vi "移动鼠标并单击.vi"(8 "错误输入（无错误）":errorcluster, 10 "dy":i32=36, 11 "dx":i32=1683) -> (0 "错误输出":errorcluster)   [LabVIEW 2012]
uses:
  User32.dll
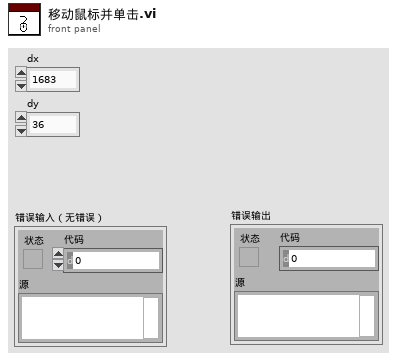
[diagram p1: front panel]
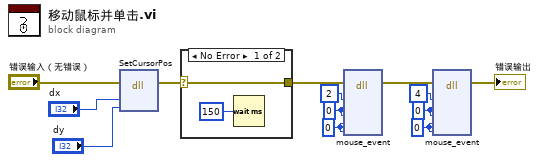
[diagram p0: block diagram]
diagram:
  w4 = 0 ("dwExtraInfo")
  w5 = u32 0 ("dwExtraInfo")
  w8 = 0 ("dwExtraInfo")
  w9 = u32 0 ("dwExtraInfo")
  n1 = dll-call lib="User32.dll" fn="SetCursorPos" ("Move mouse to new pos")(error in="错误输入（无错误）", "dx"="dx", "dy"="dy") -> (error out=w11:errorcluster)  [unwired: 5 in, 1 out]
  n2 = case shown="No Error" w11 {
    selector: w11 -> [w14 w16]
    tunnel: [w14 w16] -> w7
    frame No Error {
      n3 = Wait (ms)(milliseconds to wait=u32 150 ("等待时间（毫秒）")) -> ()  [unwired: 1 out]
    }
    frame Error {
    }
  }
  n4 = dll-call lib="user32.dll" fn="mouse_event" label="Mouse_Event"(error in=w7, "dwFlags"=2, "dx"=w8, "dy"=w8, "dwData"=w9, "dwExtraInfo"=w9) -> (error out=w3:errorcluster)  [unwired: 8 in, 1 out]
  n5 = dll-call lib="user32.dll" fn="mouse_event" label="Mouse_Event"(error in=w3, "dwFlags"=4, "dx"=w4, "dy"=w4, "dwData"=w5, "dwExtraInfo"=w5) -> (error out=→"错误输出":errorcluster)  [unwired: 8 in, 1 out]
